vi "_UTIL_Run_ExcelTest.vi"() -> ()   [LabVIEW 2024]
uses:
  Control Definitions/Def Results2.ctl
panel:
  in  "File Name 2":string="AEPS2"
  in  "Root path 2":path=path "C:/AllenProjects/PWC-OLS"
  in  "Results out 3":T1=[[{"Fill"=0.0, "Drain"=0.0, "Status"=0, "Resistor"=0.0}, {"Fill"=0.0, "Drain"=0.0, "Status"=1, "Resistor"=0.0}], [{"Fill"=0.0, "Drain"=7.5701486385059376, "Status"=9, "Resistor"=100.6449013199144}, {"Fill"=7.784591865043643, "Drain"=7.332779690256121, "Status"=9, "Resistor"=100.51621086193613}], [{"Fill"=7.484951390528681, "Drain"=7.103353498597148, "Status"=5, "Resistor"=200.93382929629374}, {"Fill"=7.27937277320862, "Drain"=6.899822595281603, "Status"=5, "Resistor"=200.88464528358477}], [{"Fill"=7.063569408888819, "Drain"=6.663750151243212, "Status"=5, "Resistor"=301.0356513903887}, {"Fill"=6.850342846689227, "Drain"=6.42888031019211, "Status"=5, "Resistor"=301.33612029506116}], [{"Fill"=6.617313850955965, "Drain"=6.212398902769091, "Status"=5, "Resistor"=401.2244680894643}, {"Fill"=6.392705221085551, "Drain"=5.995307375717164, "Status"=5, "Resistor"=401.51541036550975}], [{"Fill"=6.149188364262583, "Drain"=5.763065338974001, "Status"=5, "Resistor"=501.39150779294386}, {"Fill"=5.947703029999735, "Drain"=5.539097573041918, "Status"=5, "Resistor"=501.5781570850042}], [{"Fill"=5.7123960954332365, "Drain"=5.306385076866151, "Status"=5, "Resistor"=601.4999053941204}, {"Fill"=5.474618891353609, "Drain"=5.0769705632782, "Status"=5, "Resistor"=601.7261122344689}], [{"Fill"=5.257989243927004, "Drain"=4.862330954484942, "Status"=5, "Resistor"=701.4913550474793}, {"Fill"=5.037681719112398, "Drain"=4.629592242231371, "Status"=5, "Resistor"=701.7927309302642}], [{"Fill"=4.801631677904131, "Drain"=4.40018297185898, "Status"=5, "Resistor"=801.5996734374615}, {"Fill"=4.588669421434404, "Drain"=4.177654706926347, "Status"=5, "Resistor"=801.8507162107668}], [{"Fill"=4.333037400074007, "Drain"=3.959183737525942, "Status"=6, "Resistor"=901.7398273051579}, {"Fill"=4.139064640398027, "Drain"=3.72557608145714, "Status"=5, "Resistor"=902.0735543073872}], [{"Fill"=3.91243236764908, "Drain"=0.0, "Status"=6, "Resistor"=1002.0488441152058}, {"Fill"=3.685923072137834, "Drain"=3.7199901502609265, "Status"=10, "Resistor"=1002.0588187536472}]] {"Resistor" format="%.1f"; "Drain" format="%.3f"; "Fill" format="%.3f"}
  in  "Data Out":dbl[][](array[numeric])=array12052x6[72312 elements]
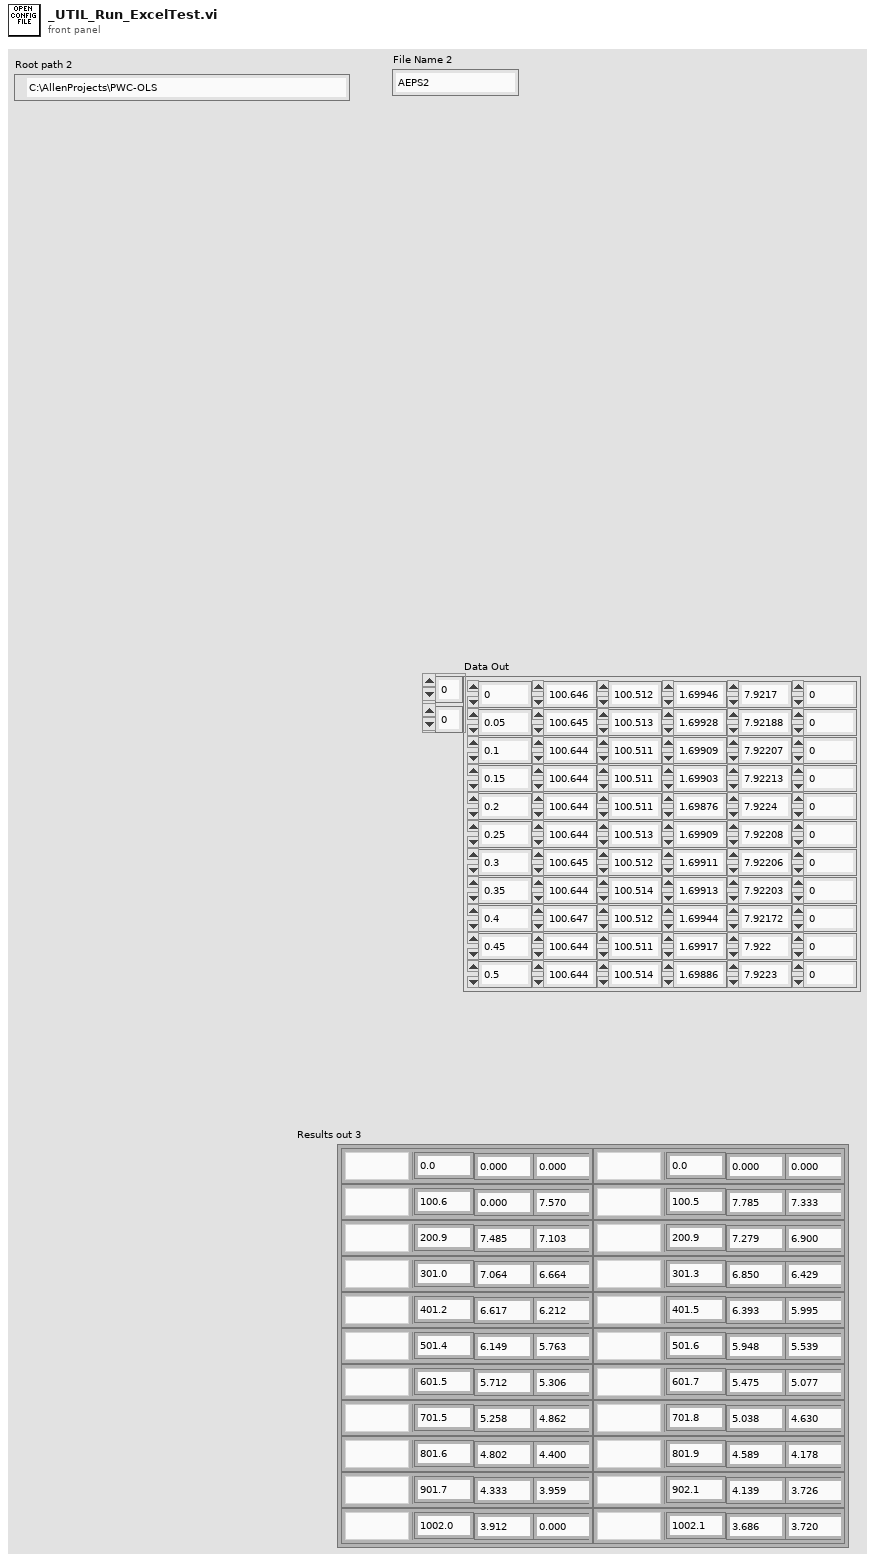
[diagram p1: front panel]
types:
  T1 = typedef "Def Results2.ctl" = cluster{"Fill":dbl, "Drain":dbl, "Status":i16, "Resistor":dbl}[][]
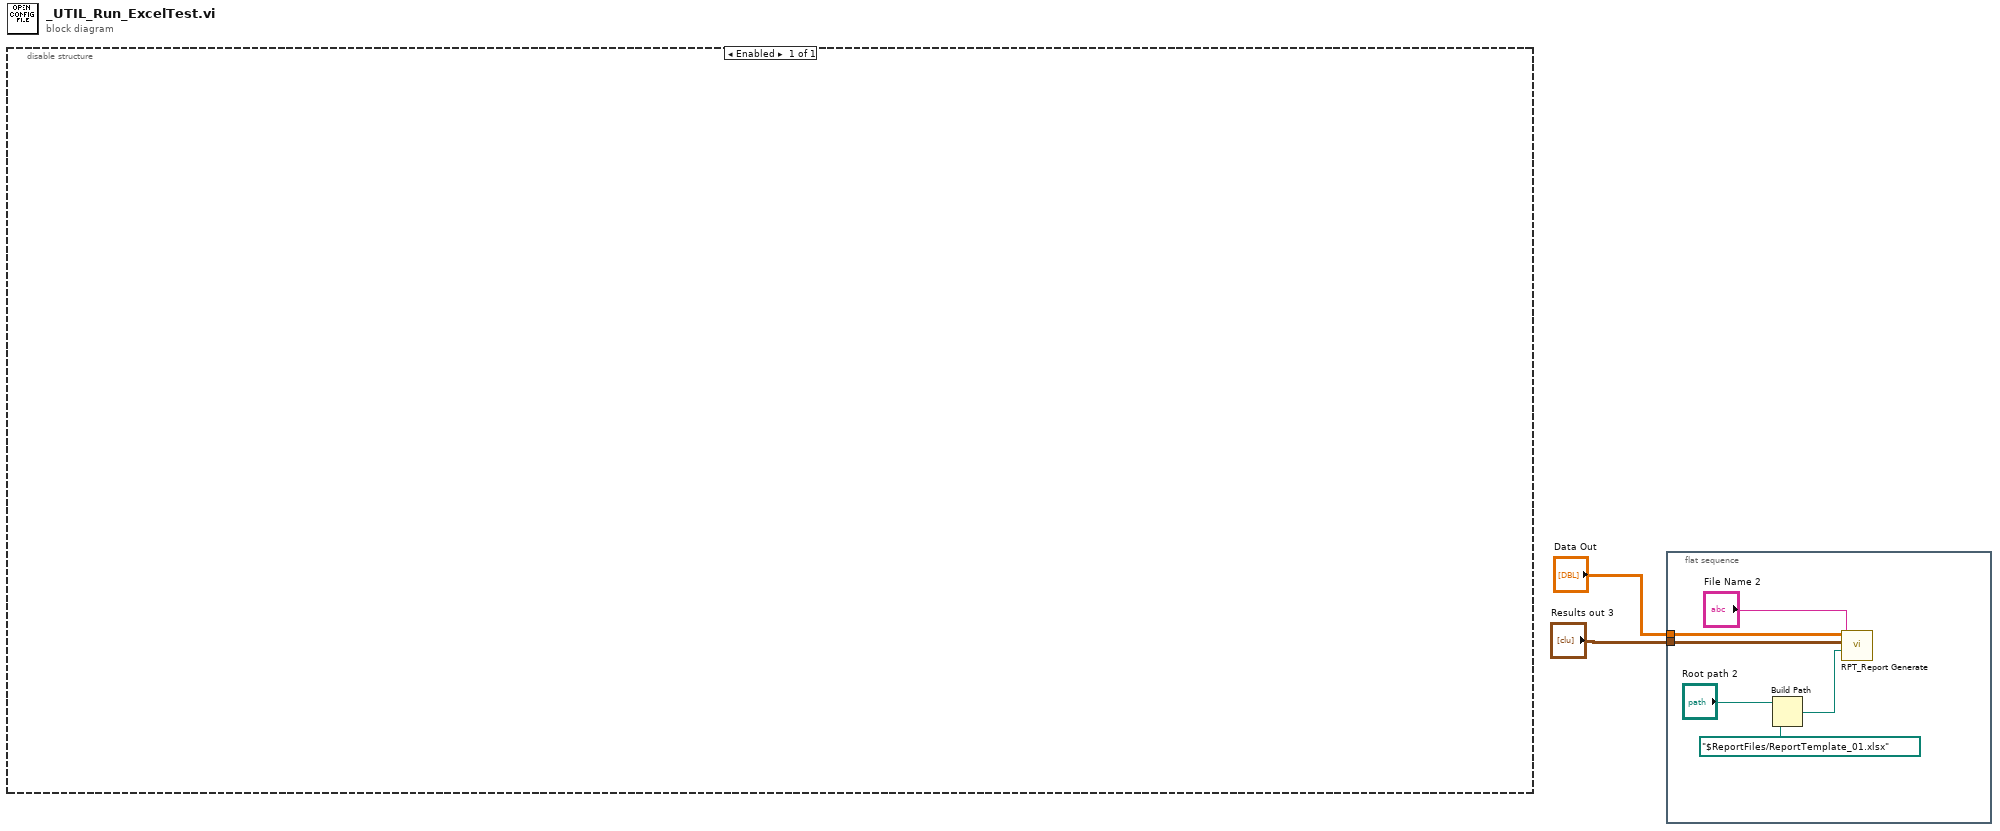
[diagram p0: block diagram]
diagram:
  n1 = disable-structure shown="Enabled" {
    frame Enabled {
    }
  }
  n2 = flat-sequence {
    tunnel: "Data Out" -> [w8]
    tunnel: "Results out 3" -> [w7]
    frame #0 {
      n3 = Build Path(base path="Root path 2", name or relative path=path "$ReportFiles/ReportTemplate_01.xlsx") -> (appended path=w5:path)
      n4 = call "RPT_Report Generate.vi"("Report Name"="File Name 2", "template"=w5, "Results"=w7, "Wave Data"=w8) -> ()  [unwired: 8 in]
    }
  }
